vi "Madelung Energy Correction.vi"(9 "Dielectric Constant":dbl=11.0, 10 "Volume (A³)":dbl=7795.605843681768, 11 "Net Charge":i32=1) -> (2 "Madelung Only correction":dbl=0.08316511317738377, 3 "1st Order correction (eV)":dbl=0.057232718795708654)   [LabVIEW 2010]
panel:
  out "Madelung constant for cubic 2":dbl
  in  "Madelung constant for cubic":dbl=2.744347059
  out "E0":dbl=0.06944616161583614
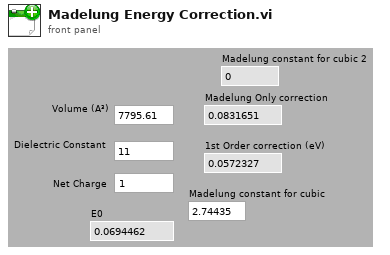
[diagram p1: front panel]
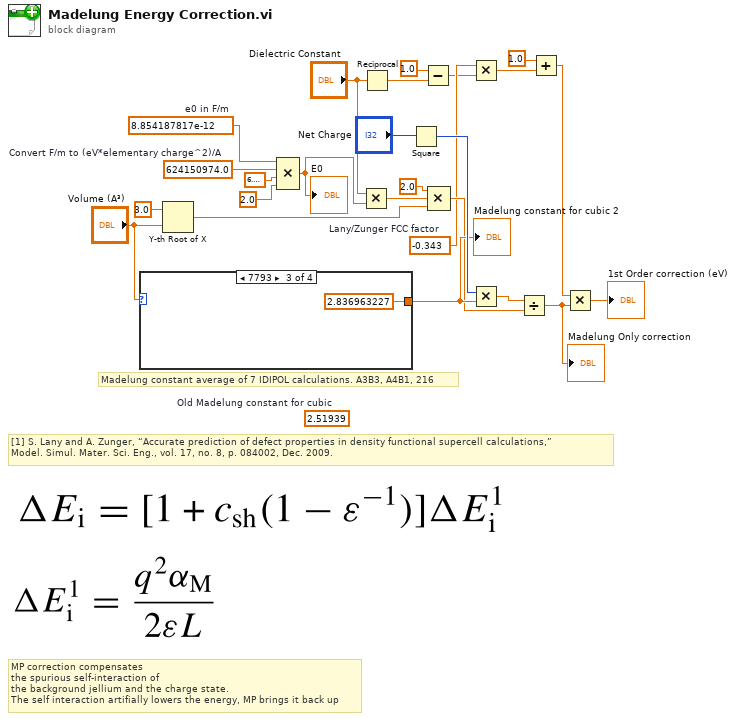
[diagram p0: block diagram]
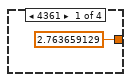
[diagram p2: hidden frame]
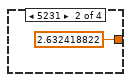
[diagram p3: hidden frame]
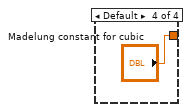
[diagram p4: hidden frame]
diagram:
  (unwired) 2.51939  # Old Madelung constant for cubic
  w15 = -0.343  # Lany/Zunger FCC factor
  w3 = 624150974.0  # Convert F/m to (eV*elementary charge^2)/A
  w4 = 8.854187817e-12  # e0 in F/m
  # "Madelung constant average of 7 IDIPOL calculations. A3B3, A4B1, 216"
  # "MP correction compensates\nthe spurious self-interaction of\nthe background jellium and the charge state.\nThe self interaction artifially lowers the energy, MP brings it back up"
  # "[1] S. Lany and A. Zunger, “Accurate prediction of defect properties in density functional supercell calculations,” \nModel. Simul. Mater. Sci. Eng., vol. 17, no. 8, p. 084002, Dec. 2009."
  n1 = case shown="7793" "Volume (A³)" {
    tunnel: [2.763659129 ("Madelung constant for cubic") 2.632418822 ("Madelung constant for cubic") 2.836963227 ("Madelung constant for cubic") "Madelung constant for cubic"] -> w23
    frame 4361 {
    }
    frame 5231 {
    }
    frame 7793 {
    }
    frame Default {
    }
  }
  "Madelung constant for cubic 2" <- w23
  n2 = Y-th Root of X(1:"Volume (A³)", 2:3.0 ("y")) -> (0:w19:dbl)
  n3 = Compound Arithmetic op=MULTIPLY(w4, w3, 6.283185307179586, 2.0 ("y")) -> (w2:dbl)
  "E0" <- w2
  n4 = Multiply(x="Dielectric Constant", y=w2) -> (x*y=w17:dbl)
  n5 = Reciprocal(x="Dielectric Constant") -> (1/x=w12:dbl)
  n6 = Square(x="Net Charge") -> (x^2=w24:i32)
  n7 = Subtract(x=1.0, y=w12) -> (x-y=w11:dbl)
  n8 = Compound Arithmetic op=MULTIPLY(2.0 ("value"), w17, w19) -> (w18:dbl)
  n9 = Multiply(x=w15, y=w11) -> (x*y=w10:dbl)
  n10 = Multiply(x=w24, y=w23) -> (x*y=w22:dbl)
  n11 = Divide(x=w22, y=w18) -> (x/y=w8:dbl)
  "Madelung Only correction" <- w8
  n12 = Add(x=1.0, y=w10) -> (x+y=w9:dbl)
  n13 = Multiply(x=w9, y=w8) -> (x*y=→"1st Order correction (eV)":dbl)
